vi "Read transfer config.vi"(8 "error in (no error)":errorcluster, 11 "Runtime.Transfer in":refnum<class "Runtime.Transfer.lvclass">) -> (0 "error out":errorcluster, 2 "transfer config":T1, 3 "Runtime.Transfer out":refnum<class "Runtime.Transfer.lvclass">)   [LabVIEW 2016, in "Data Sharing Framework.Runtime.lvlib" / "Runtime.Transfer.lvclass"]
uses:
  Runtime.Transfer.lvclass
  Typedefs/Transfer Config.ctl
  Typedefs/Transfer Direction.ctl
  Typedefs/Decimation Factors.ctl
  Runtime.Transfer.lvclass/Runtime.Transfer.ctl
  Data Sharing Framework.Configuration.lvlib
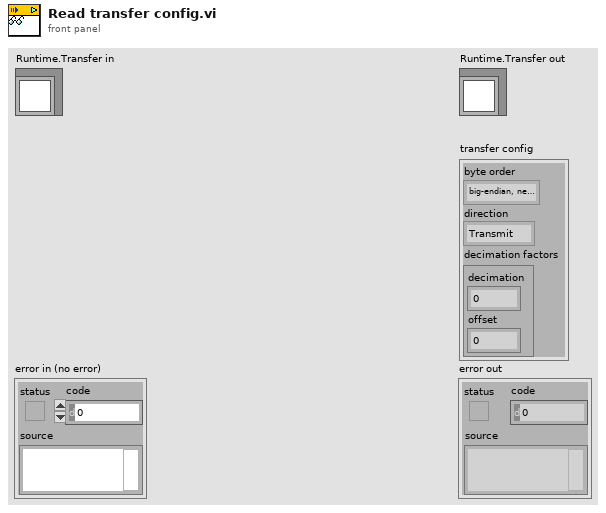
[diagram p1: front panel]
types:
  T1 = typedef "Data Sharing Framework.Configuration.lvlib/Transfer Config.ctl" = cluster{"byte order":enum16{"big-endian, network order", "native, host order", "little-endian"}, "direction":T2, "decimation factors":T3}
  T2 = typedef "Data Sharing Framework.Configuration.lvlib/Transfer Direction.ctl" = enum16{"Transmit", "Receive"}
  T3 = typedef "Data Sharing Framework.Configuration.lvlib/Decimation Factors.ctl" = cluster{"decimation":u16, "offset":u16}
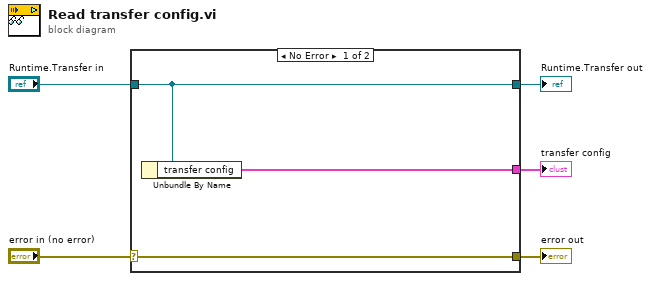
[diagram p0: block diagram]
diagram:
  n1 = case shown="No Error" "error in (no error)" {
    selector: "error in (no error)" -> [w8 w9]
    tunnel: [w8 w9] -> w4
    tunnel: [w7 w10] -> w2
    tunnel: "Runtime.Transfer in" -> [w7 w10]
    tunnel: [w6 _] -> w1
    frame No Error {
      n2 = Unbundle By Name(w7) -> ("transfer config"=w6:T1)
    }
    frame Error {
    }
  }
  "error out" <- w4
  "Runtime.Transfer out" <- w2
  "transfer config" <- w1
